vi "AddCartesianVectors.vi"(8 "error in (no error)":errorcluster, 11 "CartesianVector in A":refnum<class "CartesianVector.lvclass">) -> (0 "error out":errorcluster, 3 "CartesianVector out":refnum<class "CartesianVector.lvclass">)   [LabVIEW 2013, in "CartesianVector.lvclass"]
uses:
  CartesianVector.lvclass
  CartesianVector.lvclass/CartesianVector.ctl
panel:
  in  "CartesianVector in B":refnum<class "CartesianVector.lvclass">
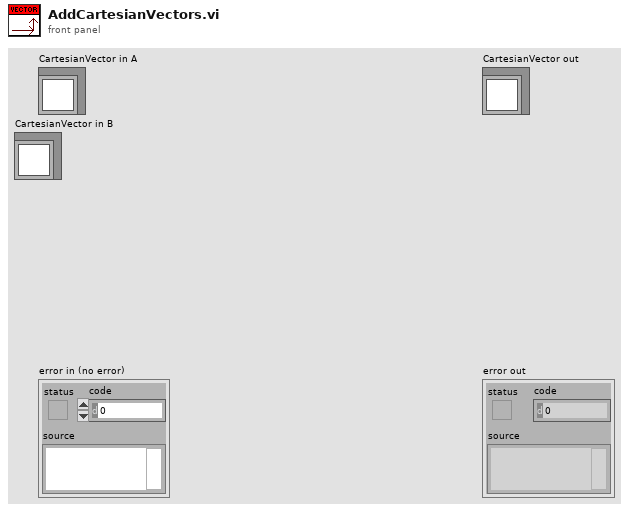
[diagram p1: front panel]
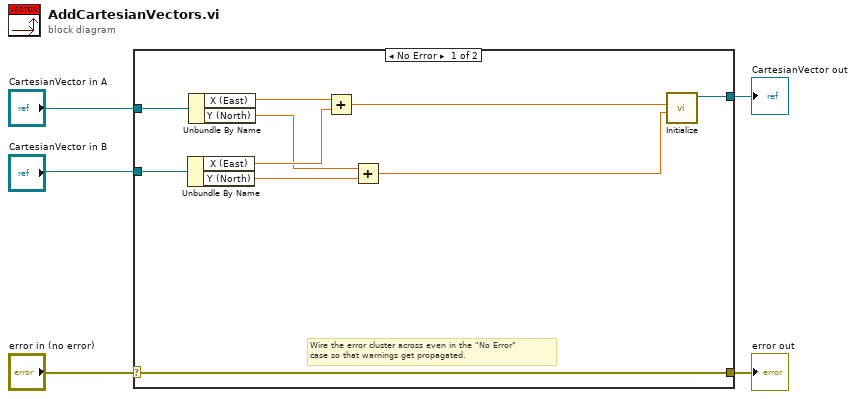
[diagram p0: block diagram]
diagram:
  n1 = case shown="No Error" "error in (no error)" {
    selector: "error in (no error)" -> [w15 w17]
    tunnel: [w15 w17] -> w4
    tunnel: [w14 w16] -> w2
    tunnel: "CartesianVector in A" -> [w13 w16]
    tunnel: "CartesianVector in B" -> [w12 _]
    frame No Error {
      # "Wire the error cluster across even in the \"No Error\"\ncase so that warnings get propagated."
      n2 = Unbundle By Name(w12) -> ("X (East)"=w10:dbl, "Y (North)"=w9:dbl)
      n3 = Unbundle By Name(w13) -> ("X (East)"=w11:dbl, "Y (North)"=w8:dbl)
      n4 = Add(x=w11, y=w10) -> (x+y=w6:dbl)
      n5 = Add(x=w8, y=w9) -> (x+y=w7:dbl)
      n6 = call "Initialize.vi"("Y (North)"=w7, "X (East)"=w6) -> ("CartesianVector out"=w14:refnum<class "CartesianVector.lvclass">)  [unwired: 8 in, 1 out]
    }
    frame Error {
    }
  }
  "error out" <- w4
  "CartesianVector out" <- w2
